vi "LM model function and gradient (1-Exp, Gated, Periodic).vi"(3 "output control":T1, 4 "data":variant, 5 "X":dbl[](array[numeric]), 6 "a":dbl[](array[numeric]) format="%_5g") -> (0 "error out":errorcluster, 1 "f'(X,a)":dbl[][](array[numeric]), 2 "f(X,a)":dbl[](array[numeric]))   [LabVIEW 2021, in "Fits.lvlib"]
doc: "This template is the starting point for creating a model function to be passed to the Nonlinear Curve Fit.vi."
uses:
  Fits.lvlib
  <vilib>/gmath/NumericalOptimization/LM_output select.ctl
  Fit Control Data.ctl
  Graphs/XY Graph/XY Graph Plot Data.ctl
  e236fd45-a14d-46c2-aa23-4f6afb79c3c8.vi
  aab2c552-8d76-4341-aab1-b49ec4ad7e74.vi
  Arrays/Threshold 1D T-Periodic Array (xN).vi/9126c8e0-c887-40cd-9668-65afecc2b031.vi
  Comparison/All X[i] ~ 0 [DBL].vi
  Arrays/Arrays.lvlib
  Utilities/Utilities.lvlib
  Graphs/XY Graph/XY Graph Add-Ons.lvlib
  <vilib>/gmath/NI_Gmath.lvlib
panel:
  out "XY Graph":cluster{"X":dbl[], dbl[]}[](graph)
  # "t0\n\nBL\n\nA1\n\ntau1"
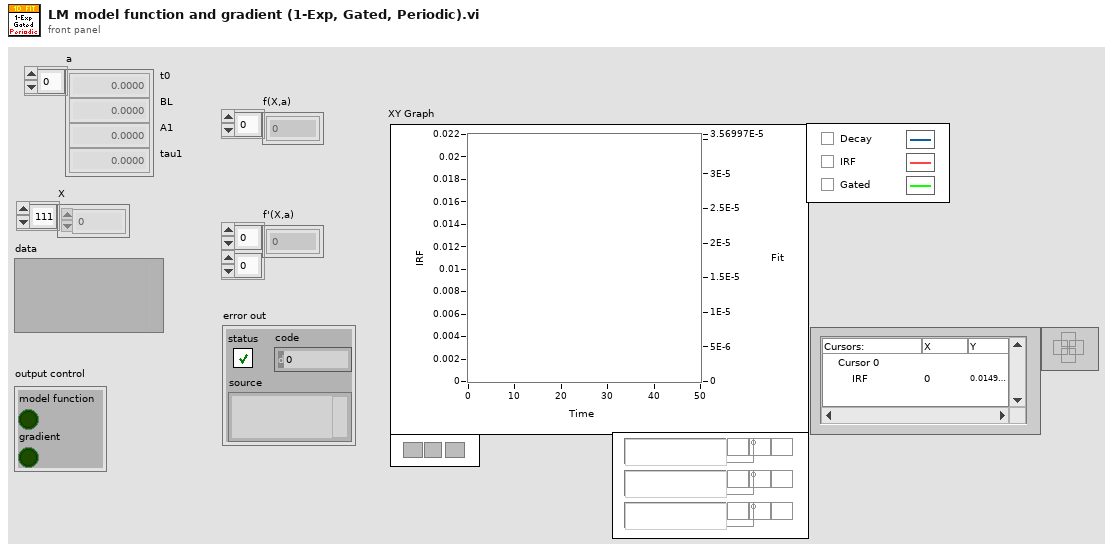
[diagram p1: front panel]
types:
  T1 = typedef "NI_Gmath.lvlib/LM_output select.ctl" = cluster{"model function":bool, "gradient":bool}
  T2 = typedef "Fits.lvlib/Fit Control Data.ctl" = cluster{"IRF":T3, "Laser Period":dbl, "SYNC Period":dbl}
  T3 = typedef "XY Graph Add-Ons.lvlib/XY Graph Plot Data.ctl" = cluster{"X Array":dbl[], "Y Array":dbl[]}
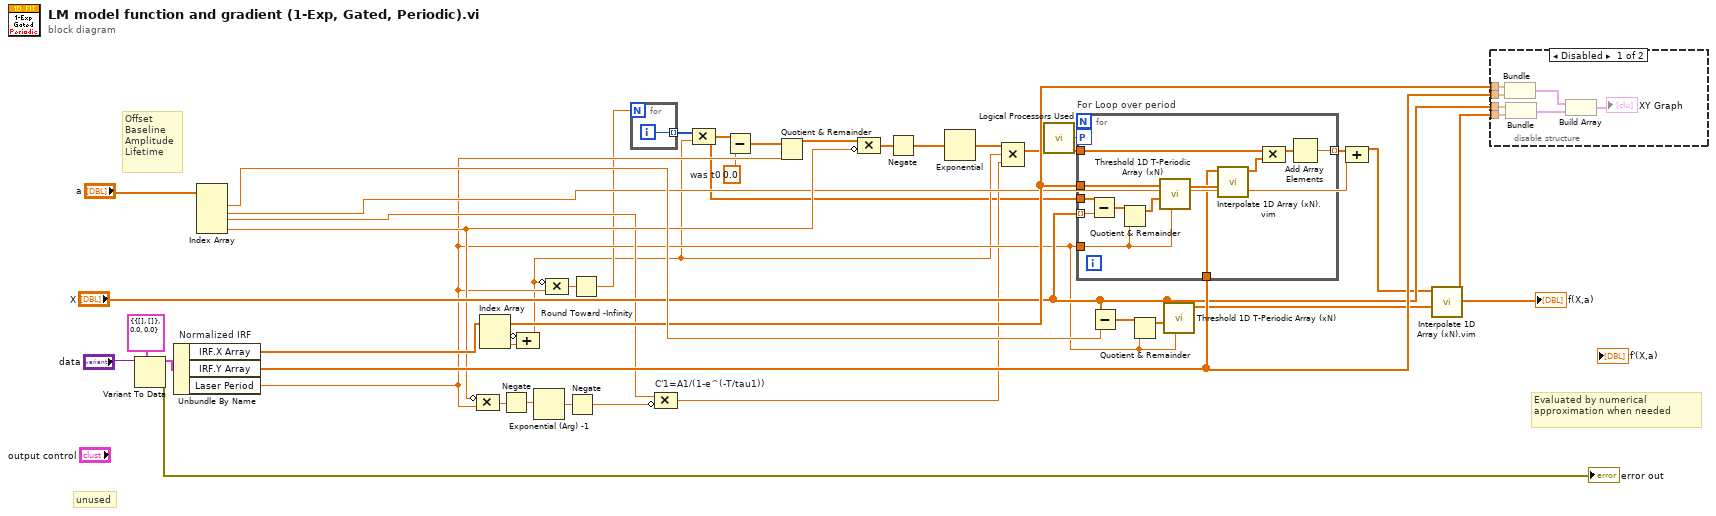
[diagram p0: block diagram]
diagram:
  w6 = 0.0  # was t0
  # "unused"
  # "Evaluated by numerical approximation when needed"
  # "Offset\nBaseline\nAmplitude\nLifetime"
  n1 = Variant To Data(type=T2 {"IRF"={"X Array"=[], "Y Array"=[]}, "Laser Period"=0.0, "SYNC Period"=0.0} ("Fit Control Data"), Variant="data") -> (data=w37:T2, error out=→"error out":errorcluster)  [unwired: 1 in]
  n2 = Unbundle By Name "Normalized IRF"(w37) -> ("IRF.X Array"=w32:dbl[], "IRF.Y Array"=w33:dbl[], "Laser Period"=w26:dbl)
  n3 = Index Array(array="a") -> (element #1=w35:dbl, element #2=w27:dbl, element #3=w28:dbl, element #4=w29:dbl)  [unwired: 4 in]
  n4 = Compound Arithmetic op=MULTIPLY(invert w29, w26) -> (w24:dbl)
  n5 = Index Array(array=w32) -> (element #1=w15:dbl, element #2=w14:dbl)  [unwired: 2 in]
  n6 = Negate(x=w24) -> (-x=w23:dbl)
  n7 = Compound Arithmetic op=ADD(invert w15, w14) -> (w11:dbl)
  n8 = Exponential (Arg) -1(1:w23) -> (0:w16:dbl)
  n9 = Compound Arithmetic op=MULTIPLY(invert w11, w26) -> (w25:dbl)
  n10 = Negate(x=w16) -> (-x=w22:dbl)
  n11 = Round Toward -Infinity(1:w25) -> (0:w21:dbl)
  n12 = for {
    N: w21 -> [_]
    tunnel: [w40] -> w20 mode=indexing
    i -> [w40]
  }
  n13 = Compound Arithmetic op=MULTIPLY "C'1=A1/(1-e^(-T/tau1))"(w28, invert w22) -> (w10:dbl)
  n14 = Compound Arithmetic op=MULTIPLY(w20, w11) -> (w9:dbl[])
  n15 = Subtract(x=w9, y=w6) -> (x-y=w13:dbl[])
  n16 = Quotient & Remainder(x=w13, y=w26) -> (x-y*floor(x/y)=w12:dbl[])  [unwired: 1 out]
  n17 = Compound Arithmetic op=MULTIPLY(w12, invert w29) -> (w19:dbl[])
  n18 = Negate(x=w19) -> (-x=w7:dbl[])
  n19 = Exponential(1:w7) -> (0:w18:dbl[])
  n20 = Compound Arithmetic op=MULTIPLY(w18, w11, w10) -> (w17:dbl[])
  n21 = call "Logical Processors Used.vi"() -> ("# Logical Processor Used"=w1:i32)  [unwired: 6 in]
  n22 = for "For Loop over period" {
    tunnel: w17 -> [w43]
    tunnel: w9 -> [w51]
    tunnel: "X" -> [w50] mode=indexing
    tunnel: w26 -> [w41]
    tunnel: w33 -> [w47]
    tunnel: w32 -> [w46]
    tunnel: [w42] -> w8 mode=indexing
    workers-P: w1 -> [_]
    n23 = Subtract(x=w51, y=w50) -> (x-y=w49:dbl[])
    n24 = Quotient & Remainder(x=w49, y=w41) -> (x-y*floor(x/y)=w48:dbl[])  [unwired: 1 out]
    n25 = call "Threshold 1D T-Periodic Array (xN).vi"("Period"=w41, "Search Values"=w48, "X"=w46) -> ("Interpolated Indices"=w52:dbl[])  [unwired: 8 in]
    n26 = call "Interpolate 1D Array (xN).vim"("Interpolated Indices"=w52, "Y"=w47) -> ("Interpolated Y"=w45:dbl[])  [unwired: 9 in]
    n27 = Compound Arithmetic op=MULTIPLY(w43, w45) -> (w44:dbl[])
    n28 = Add Array Elements(numeric array=w44) -> (sum=w42:dbl)
  }
  n29 = Subtract(x="X", y=w35) -> (x-y=w5:dbl[])
  n30 = Quotient & Remainder(x=w5, y=w26) -> (x-y*floor(x/y)=w4:dbl[])  [unwired: 1 out]
  n31 = call "Threshold 1D T-Periodic Array (xN).vi"("Period"=w26, "Search Values"=w4, "X"="X") -> ("Interpolated Indices"=w3:dbl[])  [unwired: 8 in]
  n32 = Compound Arithmetic op=ADD(w8, w27) -> (w2:dbl[])
  n33 = call "Interpolate 1D Array (xN).vim"("Interpolated Indices"=w3, "Y"=w2) -> ("Interpolated Y"=w34:dbl[])  [unwired: 9 in]
  "f(X,a)" <- w34
  n34 = disable-structure shown="Disabled" {
    disable-tunnel: w34 -> [w59 _]
    disable-tunnel: w33 -> [w57 _]
    disable-tunnel: w32 -> [w56 _]
    disable-tunnel: "X" -> [w55 _]
    frame Disabled {
      n35 = Bundle("X Array"=w56, "Y Array"=w57) -> (w58:cluster{"X Array":dbl[], "Y Array":dbl[]})  [unwired: 1 in]
      n36 = Bundle("X"=w55, "Interpolated Y"=w59) -> (w54:cluster{"X":dbl[], "Interpolated Y":dbl[]})  [unwired: 1 in]
      n37 = Build Array(w58, w54) -> (→"XY Graph":cluster{"X":dbl[], "Interpolated Y":dbl[]}[])
    }
    frame Enabled {
    }
  }
